vi "Start Condition - Saturation Time (SubVI).vi"(8 "error in (no error)":errorcluster, 9 "Time":dbl, 10 "Select":i32, 11 "Cluster in":T1 {"M Event" items=["Stop", "Running", "PID", "Up Limit", "Down Limit", "Load Limit"]; "Test Type" items=["Please Select", "Triaxial Shear", "Triaxial UU", "Shearbox", "Permeability", "Consolidation (Stepped Loading)/Swelling", "Saturation (Incremental)", "User Defined", "UCT", "Isotropic Consolidation", "Swelling Pressure"]; "Data"."Test Type" items=["Please Select", "Triaxial Shear", "Triaxial UU", "Shearbox", "Permeability", "Consolidation (Stepped Loading)/Swelling", "Saturation (Incremental)", "User Defined", "UCT", "Isotropic Consolidation", "Swelling Pressure"]}) -> (0 "error out":errorcluster, 3 "Cluster out":T1 {"M Event" items=["Stop", "Running", "PID", "Up Limit", "Down Limit", "Load Limit"]; "Test Type" items=["Please Select", "Triaxial Shear", "Triaxial UU", "Shearbox", "Permeability", "Consolidation (Stepped Loading)/Swelling", "Saturation (Incremental)", "User Defined", "UCT", "Isotropic Consolidation", "Swelling Pressure"]; "Data"."Test Type" items=["Please Select", "Triaxial Shear", "Triaxial UU", "Shearbox", "Permeability", "Consolidation (Stepped Loading)/Swelling", "Saturation (Incremental)", "User Defined", "UCT", "Isotropic Consolidation", "Swelling Pressure"]})   [LabVIEW 2019]
uses:
  Controls/RunTest - Data Structure.ctl
  Controls/Test Panel - Data Structure.ctl
  Controls/Station - Test Type.ctl
  <vilib>/Utility/miscctls.llb/LVRowAndColumnTypeDef.ctl
  Controls/RunTest - Calculate Data.ctl
  <vilib>/httpClient/ClientHandle.ctl
  Controls/RunTest - Start Condition.ctl
  Controls/RunTest - Stop Condition.ctl
  Controls/UDP - Event.ctl
  <vilib>/httpClient/LabVIEWHTTPClient.lvlib
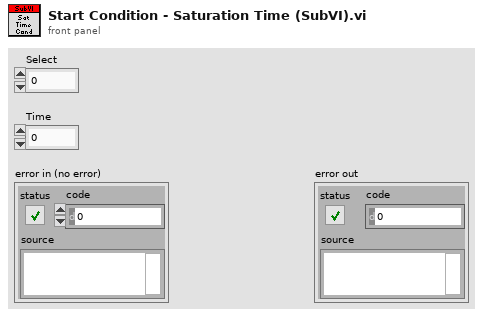
[diagram p1: front panel]
types:
  T1 = typedef "RunTest - Data Structure.ctl" = cluster{"Test Plan":string[], "PlanRow":i32, "Device Name":string[], "Timeout":i32, "Start?":bool, "Pause?":bool, "IP Address":string[], "LogRow":i32, "Logtype":u16, "Log Elapse":sgl, "Data":T2, "Stop log?":bool, "tdms":refnum<k34>, "Sensor Data":sgl[], "Start time":timestamp, "Prev Log Elapse":u32, "Plot":u16, "X-Axis":u16[], "Y-Axis":u16[], "XY":cluster{"X":dbl, "Y":dbl}[][], "End Stage?":bool, "1run":bool, "Condition":u16[], "Start Con":bool, "Log Con":bool, "Stop Con":bool, "Start Elapse":dbl, "Start Load":dbl, "Motor":i32, "StartRow":i32, "number log":i32, "Dir":bool, "Start time test":timestamp, "Auto":bool, "Check return?":bool, "Inv":cluster{"M":i32[], "Bool":bool[]}, "tdms temp":refnum<k34>, "Zero?":bool, "Plot Timer":dbl, "1st Run":bool, "TDMS Path":path, "MaxLoad":dbl, "Log Timer":sgl[], "Test Type":T3, "Log Sensor":string[], "Save?":bool, "1st Log":bool, "Y-Axis 2":u16[], "On Y-Axis 2":bool, "Decimal":u8[], "Init":cluster{"PWP TS":sgl, "Load TS":sgl, "Volume TS":sgl, "Disp TS":sgl, "CP":sgl, "Vol In":sgl, "Vol Out":sgl, "Load UCT":sgl, "Disp UCT":sgl, "PWP Sat":sgl, "CP Sat":sgl, "Volume IsoCons":sgl, "PWP IsoCons":sgl, "PWP TUU":sgl, "Load TUU":sgl, "Volume TUU":sgl, "Disp TUU":sgl, "Load Cons":sgl, "Disp Cons":sgl, "Volume Sat":sgl, "Vertical Load SB":sgl, "Vertical Disp SB":sgl, "H Disp SB":sgl, "H Load SB":sgl}, "Calc":T5, "Device Index":i32[], "Channel Index":i32[], "http ref":T6, "fileid":string, "Step Cons":cluster{"V Stress":sgl, "H Settlement":sgl}, "RunTest":bool, "Graph Last":i32, "Init?":bool, "Datalog":bool[], "Start":T7, "Stop":T8, "Running?":bool, "StartTime":dbl, "Log Prev Time":dbl, "KeyName":string[], "Test RunTime":dbl, "Log Prev Axial":dbl, "M Event":T9[], "Last Log":bool, "popup":bool, "PreStart UU":bool, "PreStart Sat":bool}
  T2 = typedef "Test Panel - Data Structure.ctl" = cluster{"Station":string, "Sample ID":string, "Job No":string, "Job Description":string, "Filename":string, "Test Type":T3, "Speciment No":string, "Depth":string, "Height":string, "Diameter/Length":string, "Weight":string, "Test Parameter":string, "Station[]":string[], "Edit Pos":T4, "Edit Pos Prev":T4, "Area":string, "Path":string}
  T3 = typedef "Station - Test Type.ctl" = u16
  T4 = typedef "LVRowAndColumnTypeDef.ctl" = cluster{"Row":i32, "Column":i32}
  T5 = typedef "RunTest - Calculate Data.ctl" = cluster{"TS":cluster{"Change PWP":sgl, "Change Vol":sgl, "Axial Load":sgl, "CiL":sgl, "Deviator":sgl, "Axial Strain":sgl, "MaxDeviator":sgl}, "TUU":cluster{"Change PWP":sgl, "Axial Load":sgl, "CiL":sgl, "Deviator":sgl, "Axial Strain":sgl, "MaxDeviator":sgl}, "Sat":cluster{"B Value":sgl, "PWP Diss":sgl, "CPP":sgl, "CV":sgl}, "Per":cluster{"Change Vol In":sgl, "Change Vol Out":sgl, "Mean Vol":sgl, "Gradient Pressure":sgl, "Outlet Flow":sgl, "Inlet Flow":sgl, "I X1":sgl, "I X2":sgl, "I Y1":sgl, "I Y2":sgl, "O X1":sgl, "O X2":sgl, "O Y1":sgl, "O Y2":sgl}, "Step Cons":cluster{"V Stress":sgl, "H Settlement":sgl, "Total H Settle":sgl, "Prev Total H":sgl}, "UCT":cluster{"ALC":sgl, "H Change":sgl, "Deviator":sgl, "Axial Strain":sgl, "V Stress":sgl, "MaxDeviator":sgl}, "ISO Cons":cluster{"CPP":sgl, "PWP Diss":sgl, "CV":sgl}, "SB":cluster{"Speci LenC":sgl, "Shear Strain":sgl, "H LC":sgl, "Normal Stress":sgl, "Shear Stress":sgl, "MaxShear":sgl}}
  T6 = typedef "LabVIEWHTTPClient.lvlib/ClientHandle.ctl" = refnum<k1>
  T7 = typedef "RunTest - Start Condition.ctl" = cluster{"Cons":cluster{"VS":dbl, "Delay":bool, "No Delay":dbl}, "Sat":cluster{"CP":dbl, "BP":dbl, "StartBP":bool, "Target CP":bool, "Target BP":bool}, "Iso":cluster{"Select":dbl, "BP":dbl, "IC2":dbl, "IC3":dbl, "IC4":dbl, ". IC6":bool, "IC6":dbl, "IC6-2":dbl, "Target":bool, "Time Cond":dbl, "Last PWP":dbl}, "TS":cluster{"SS":dbl, "Engage":bool, "ES":dbl, "LC":dbl, "PreStart":bool, "Trig SS":bool, "Drain":dbl}, "TUU":cluster{"SS":dbl, "Engage":bool, "ES":dbl, "LC":dbl, "PreStart":bool, "Trig SS":bool, "CP":dbl, "Delay Value":dbl, "Delay":bool, "CP PID":bool}, "UCT":cluster{"SS":dbl, "Engage":bool, "ES":dbl, "LC":dbl, "PreStart":bool, "Trig SS":bool}, "Enable?":bool, "SB":cluster{"SS":dbl, "Engage":bool, "ES":dbl, "LC":dbl, "PreStart":bool, "Trig SS":bool, "VS":dbl, "Delay Value":dbl, "Delay":bool, "VS PID":bool}, "Perm":cluster{"DP":dbl}}
  T8 = typedef "RunTest - Stop Condition.ctl" = cluster{"Cons":cluster{"Select":i32, "Disp":dbl, "Time":dbl, "Time2":dbl, "Disp 2":dbl, "Time Cond":dbl, "Last Disp":dbl, "Swell":bool}, "Sat":cluster{"Select":i32, "PP":dbl, "Time":dbl, "VC":dbl, "Time2":dbl, "Time Cond":dbl, "Last PP":dbl, ".B":bool, "B":dbl, "Last Vc":dbl, "Time Cond 2":dbl, "Time3":dbl, "Time Cond 3":dbl, "B Achieve":bool}, "Iso":cluster{"PP":dbl, "Time":dbl, "VC":dbl, "Time2":dbl, "Time Cond":dbl, "Last Vc":dbl, ".PP":bool, "Time Cond 2":dbl, "Select":i32}, "TS":cluster{"Axial":dbl, ".MaxDev":bool, "MaxDev Value":dbl, "Return":bool, "Reset":bool, "Prev Time":dbl, "PostStop Run":bool, "CP Stop":bool, "BP Stop":bool, "PostStop Trig":bool, "Reset Value":dbl, "BPTrig":bool, "CPTrig":bool, "VLCTrig":bool}, "TUU":cluster{"Axial":dbl, ".MaxDev":bool, "MaxDev Value":dbl, "Return":bool, "Reset":bool, "Prev Time":dbl, "PostStop Run":bool, "CP Stop":bool, "BP Stop":bool, "PostStop Trig":bool, "Reset Value":dbl, "BPTrig":bool, "CPTrig":bool, "VLCTrig":bool}, "UCT":cluster{"Axial":dbl, ".MaxDev":bool, "MaxDev Value":dbl, "Return":bool, "Reset":bool, "Prev Time":dbl, "PostStop Run":bool, "CP Stop":bool, "BP Stop":bool, "PostStop Trig":bool}, "Enable?":bool, "SB":cluster{"Shear":dbl, ".MaxShear":bool, "MaxShear Value":dbl, "Return":bool, "Reset":bool, "Prev Time":dbl, "PostStop Run":bool, "CP Stop":bool, "BP Stop":bool, "PostStop Trig":bool, "Reset Value":dbl, "BPTrig":bool, "CPTrig":bool, "VLCTrig":bool}, "Perm":cluster{"Max Time":bool, "Reset":bool, "PostStop Run":bool, "Ratio":bool, "Reset Value":dbl, "Time":dbl, "RatioTime":dbl, "RatioMore":dbl, "RatioLess":dbl, "Time Cond":dbl, "Time Cond 2":dbl, "Prev IF":dbl, "Prev OF":dbl, "PostStop Trig":bool, "BP Trig":bool, "DP Stop":bool, "BP Stop":bool, "CP Stop":bool, "CP Trig":bool}, "SP":cluster{".Max Time":bool, ".Time":bool, "Time":dbl, "MaxTime":dbl, "Time Cond":dbl, "Max Time Cond":dbl, "Stress":dbl}}
  T9 = typedef "UDP - Event.ctl" = u16
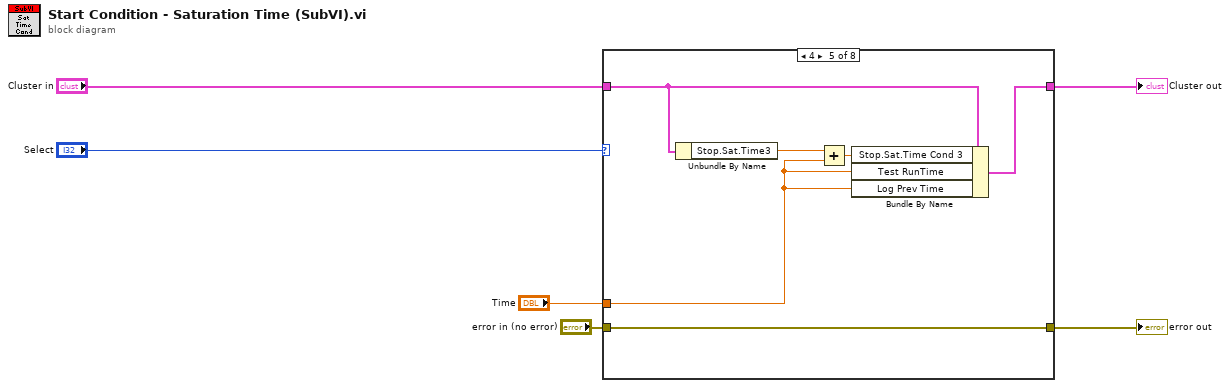
[diagram p0: block diagram]
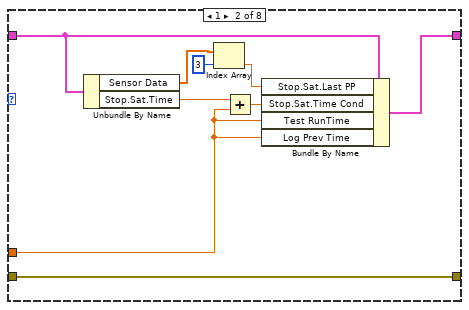
[diagram p3: hidden frame]
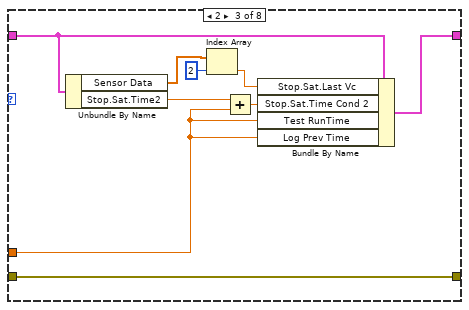
[diagram p4: hidden frame]
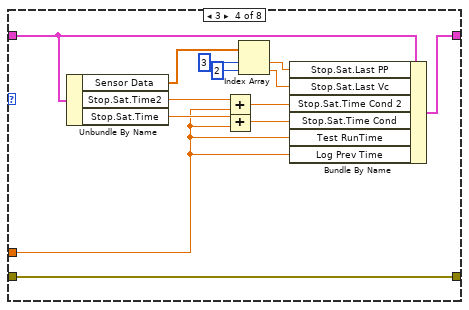
[diagram p5: hidden frame]
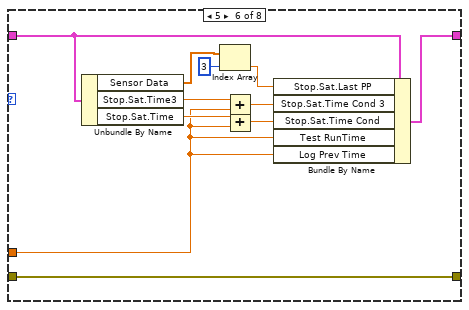
[diagram p6: hidden frame]
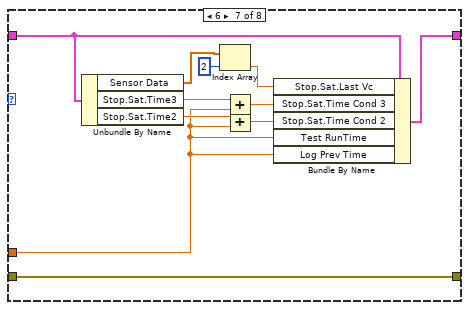
[diagram p7: hidden frame]
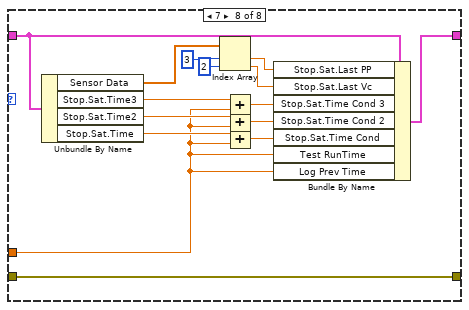
[diagram p8: hidden frame]
diagram:
  n1 = case shown="4" "Select" {
    tunnel: "Time" -> [_ w13 w22 w27 w41 w46 w57 w69]
    tunnel: [w7 w17 w26 w39 w45 w56 w67 w82] -> w1
    tunnel: "Cluster in" -> [w7 w15 w24 w37 w43 w54 w65 w81]
    tunnel: [w8 w9 w18 w32 w40 w52 w63 w79] -> w5
    tunnel: "error in (no error)" -> [w8 w9 w18 w32 w40 w52 w63 w79]
    frame Default {
    }
    frame 1 {
      n2 = Unbundle By Name(w15) -> ("Sensor Data"=w11:sgl[], "Stop.Sat.Time"=w14:dbl)
      n3 = Index Array(array=w11, index=3) -> (element=w10:sgl)
      n4 = Add(x=w14, y=w13) -> (x+y=w16:dbl)
      n5 = Bundle By Name(cluster=w15, "Stop.Sat.Last PP"=w10, "Stop.Sat.Time Cond"=w16, "Test RunTime"=w13, "Log Prev Time"=w13) -> (w17:T1)
    }
    frame 2 {
      n6 = Unbundle By Name(w24) -> ("Sensor Data"=w20:sgl[], "Stop.Sat.Time2"=w23:dbl)
      n7 = Index Array(array=w20, index=2) -> (element=w19:sgl)
      n8 = Add(x=w23, y=w22) -> (x+y=w25:dbl)
      n9 = Bundle By Name(cluster=w24, "Stop.Sat.Last Vc"=w19, "Stop.Sat.Time Cond 2"=w25, "Test RunTime"=w22, "Log Prev Time"=w22) -> (w26:T1)
    }
    frame 3 {
      n10 = Unbundle By Name(w37) -> ("Sensor Data"=w34:sgl[], "Stop.Sat.Time2"=w36:dbl, "Stop.Sat.Time"=w28:dbl)
      n11 = Add(x=w36, y=w27) -> (x+y=w38:dbl)
      n12 = Add(x=w28, y=w27) -> (x+y=w29:dbl)
      n13 = Index Array(array=w34, index #1=3 ("index"), index #2=2 ("index")) -> (element #1=w30:sgl, element #2=w33:sgl)
      n14 = Bundle By Name(cluster=w37, "Stop.Sat.Last PP"=w30, "Stop.Sat.Last Vc"=w33, "Stop.Sat.Time Cond 2"=w38, "Stop.Sat.Time Cond"=w29, "Test RunTime"=w27, "Log Prev Time"=w27) -> (w39:T1)
    }
    frame 4 {
      n15 = Unbundle By Name(w43) -> ("Stop.Sat.Time3"=w42:dbl)
      n16 = Add(x=w42, y=w41) -> (x+y=w44:dbl)
      n17 = Bundle By Name(cluster=w43, "Stop.Sat.Time Cond 3"=w44, "Test RunTime"=w41, "Log Prev Time"=w41) -> (w45:T1)
    }
    frame 5 {
      n18 = Unbundle By Name(w54) -> ("Sensor Data"=w50:sgl[], "Stop.Sat.Time3"=w53:dbl, "Stop.Sat.Time"=w47:dbl)
      n19 = Index Array(array=w50, index=3) -> (element=w49:sgl)
      n20 = Add(x=w53, y=w46) -> (x+y=w55:dbl)
      n21 = Add(x=w47, y=w46) -> (x+y=w48:dbl)
      n22 = Bundle By Name(cluster=w54, "Stop.Sat.Last PP"=w49, "Stop.Sat.Time Cond 3"=w55, "Stop.Sat.Time Cond"=w48, "Test RunTime"=w46, "Log Prev Time"=w46) -> (w56:T1)
    }
    frame 6 {
      n23 = Unbundle By Name(w65) -> ("Sensor Data"=w61:sgl[], "Stop.Sat.Time3"=w64:dbl, "Stop.Sat.Time2"=w58:dbl)
      n24 = Index Array(array=w61, index=2) -> (element=w60:sgl)
      n25 = Add(x=w64, y=w57) -> (x+y=w66:dbl)
      n26 = Add(x=w58, y=w57) -> (x+y=w59:dbl)
      n27 = Bundle By Name(cluster=w65, "Stop.Sat.Last Vc"=w60, "Stop.Sat.Time Cond 3"=w66, "Stop.Sat.Time Cond 2"=w59, "Test RunTime"=w57, "Log Prev Time"=w57) -> (w67:T1)
    }
    frame 7 {
      n28 = Unbundle By Name(w81) -> ("Sensor Data"=w77:sgl[], "Stop.Sat.Time3"=w80:dbl, "Stop.Sat.Time2"=w72:dbl, "Stop.Sat.Time"=w70:dbl)
      n29 = Index Array(array=w77, index #1=3 ("index"), index #2=2 ("index")) -> (element #1=w73:sgl, element #2=w76:sgl)
      n30 = Add(x=w80, y=w69) -> (x+y=w71:dbl)
      n31 = Add(x=w72, y=w69) -> (x+y=w75:dbl)
      n32 = Add(x=w70, y=w69) -> (x+y=w68:dbl)
      n33 = Bundle By Name(cluster=w81, "Stop.Sat.Last PP"=w73, "Stop.Sat.Last Vc"=w76, "Stop.Sat.Time Cond 3"=w71, "Stop.Sat.Time Cond 2"=w75, "Stop.Sat.Time Cond"=w68, "Test RunTime"=w69, "Log Prev Time"=w69) -> (w82:T1)
    }
  }
  "error out" <- w5
  "Cluster out" <- w1
